vi "Write log.vi"(8 "error in (no error)":errorcluster, 9 "Event data":string="Event data", 10 "Event":string, 11 "Log path":path) -> (0 "error out":errorcluster)   [LabVIEW 2015]
uses:
  <vilib>/Utility/file.llb/Write Delimited Spreadsheet (string).vi
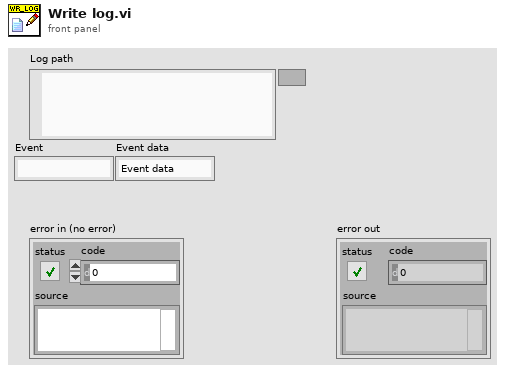
[diagram p1: front panel]
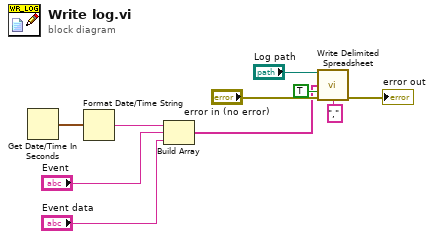
[diagram p0: block diagram]
diagram:
  n1 = Get Date/Time In Seconds() -> (seconds since 1Jan1904=w5:timestamp)
  n2 = Format Date/Time String(seconds (now)=w5) -> (date/time string=w4:string)  [unwired: 2 in]
  n3 = Build Array(w4, "Event", "Event data") -> (w3:string[])
  n4 = call-poly <vilib>:"Write Delimited Spreadsheet.vi"("file path (dialog if empty)"="Log path", "1D data"=w3, "append to file? (F)"=TRUE, "error in (no error)"="error in (no error)", "delimiter (\\t)"="," ("delimiter (\\t)")) -> ("error out"=→"error out":errorcluster)  [unwired: 9 in, 1 out]
